vi "AdvanceCurrentRepeat.vi"(8 "error in (no error)":errorcluster, 11 "RampProgramModel in":refnum<class "RampProgramModel.lvclass">) -> (0 "error out":errorcluster, 2 "EndOfRepeats":bool, 3 "RampProgramModel out":refnum<class "RampProgramModel.lvclass">)   [LabVIEW 2013, in "RampProgramModel.lvclass"]
uses:
  RampProgramModel.lvclass
  RampProgramModel.lvclass/RampProgramModel.ctl
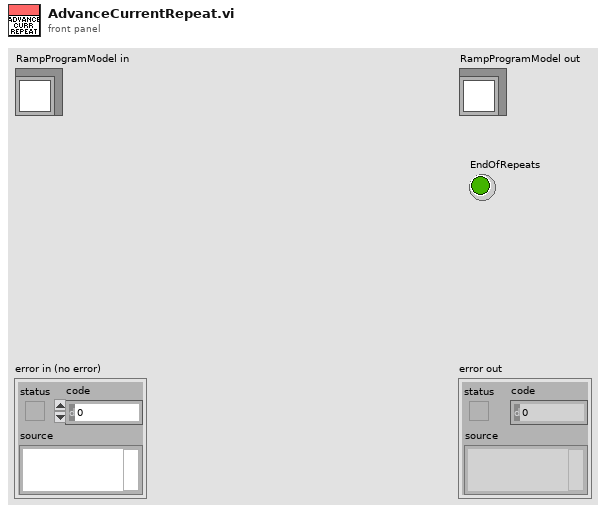
[diagram p1: front panel]
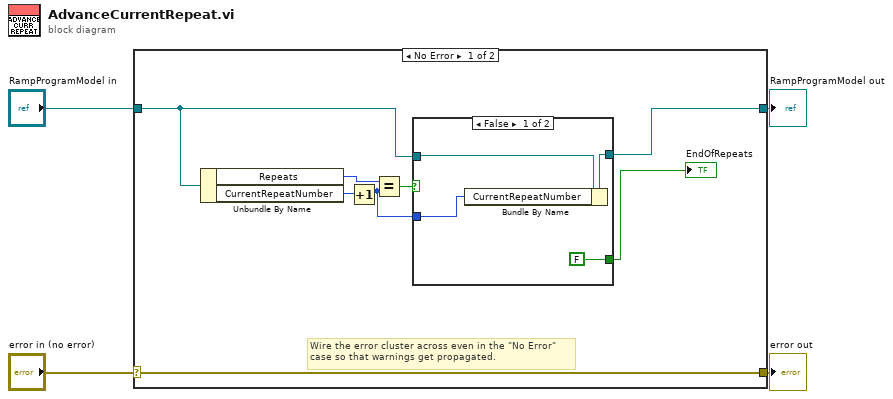
[diagram p0: block diagram]
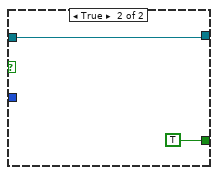
[diagram p2: hidden frame]
diagram:
  n1 = case shown="No Error" "error in (no error)" {
    selector: "error in (no error)" -> [w12 w20]
    tunnel: [w12 w20] -> w3
    tunnel: [w7 w19] -> w1
    tunnel: "RampProgramModel in" -> [w8 w19]
    frame No Error {
      # "Wire the error cluster across even in the \"No Error\"\ncase so that warnings get propagated."
      n2 = Unbundle By Name(w8) -> ("Repeats"=w11:u32, "CurrentRepeatNumber"=w6:u32)
      n3 = Increment(x=w6) -> (x+1=w5:u32)
      n4 = Equal?(x=w11, y=w5) -> (x = y?=w10:bool)
      n5 = case shown="False" w10 {
        tunnel: [FALSE ("EndOfPrograms") TRUE ("EndOfPrograms")] -> w9
        tunnel: w8 -> [w15 w17]
        tunnel: [w14 w17] -> w7
        tunnel: w5 -> [w13 _]
        frame False {
          n6 = Bundle By Name(cluster=w15, "CurrentRepeatNumber"=w13) -> (w14:refnum<class "RampProgramModel.lvclass">)
        }
        frame True {
        }
      }
      "EndOfRepeats" <- w9
    }
    frame Error {
    }
  }
  "error out" <- w3
  "RampProgramModel out" <- w1
